vi "Automatic-Approach-Retraction-MCL-2013-04-28-1a-data-storage.vi"() -> ()   [LabVIEW 2012]
uses:
  <vilib>/rvi/eio/common/nirviEmuTemplateMethod_errors.vi
  <vilib>/rvi/Emulation/niFpgaSctlEmulationGetInTimedLoop.vi
  <vilib>/rvi/Emulation/niFpgaSctlEmulationGlobalWrite.vi
  <vilib>/rvi/interface/RandomDataEmulation/nirviRandomDataFPGAFIFO.vi
  <vilib>/rvi/interface/RandomDataEmulation/niFpgaRandomDataHandleErrors.vi
  <vilib>/eio/EIONode/EIONode.xnode
  <vilib>/rvi/Analysis/measure/butterworth/XNode/niFpgaButterworthFilter.xnode
  <vilib>/rvi/DataTransferAndStorage/Container/XNode/niFpgaContainer.xnode
  <vilib>/rvi/interface/RandomDataEmulation/nirviRandomDataFpgaReadWriteTemplate.vi
panel:
  out "Tick Count(Ticks)":u32=3198398528
  in  "Data Acquisition Rate (usec)":u32=500000
  out "Data storage":bool=TRUE
  in  "Safetip Control ON/Off":bool
  out "Start Approach indicator":bool
  in  "safetip time wait":u32 caption="Count(uSec)"
  in  "Safetip retraction":u16
  out "safetip minimum indicator":bool
  out "Data counter":u16
  out "Counter Output":i16
  in  "Initial Position":i16
  in  "phase 1 control":bool
  in  "Manual Control":bool
  in  "Zposition MCL fine 2":i16
  in  "MCL counter 2":u16
  out "Curve indicator":u16
  in  "Number of curves":u16
  out "TF Freq shift":i16
  out "USBS Amplitude":i16
  in  "Timeout FIFO":i32=-1
  in  "Safetip Minimum":i16
  out "Phase 2":bool
  in  "Parameter":i16
  out "Phase 1":bool
  in  "Start Approach":bool
  out "MCL counter in range?":bool
  in  "Wait-tip-before-new-approach (usec)":u32
  in  "Fast Retraction After Cycle":i32
  in  "Wait-tip-before-approach":u32
  in  "Fast Retraction before approach":i32
  in  "Offset for Fast Approach":i16
  in  "Fast Approach (usec)":u32
  out "USBS Phase Signal":i16
  in  "Minimum for Approach Value":i16
  out "digital steps per region":u16
  in  "MCL Divisions":u16
  in  "MCL counter":u16
  in  "Fine Retraction (usec)":u32
  in  "TF at infinity":i16
  out "TF Phase Signal":i16(graph)
  out "Control Signal":i16
  out "MCL Sensor":i16
  in  "Fine Approach (usec)":u32
  in  "Setpoint Fine":i16
  out "Zposition MCL fine":i16
  in  "Initial Height (Fine)":i16=9113
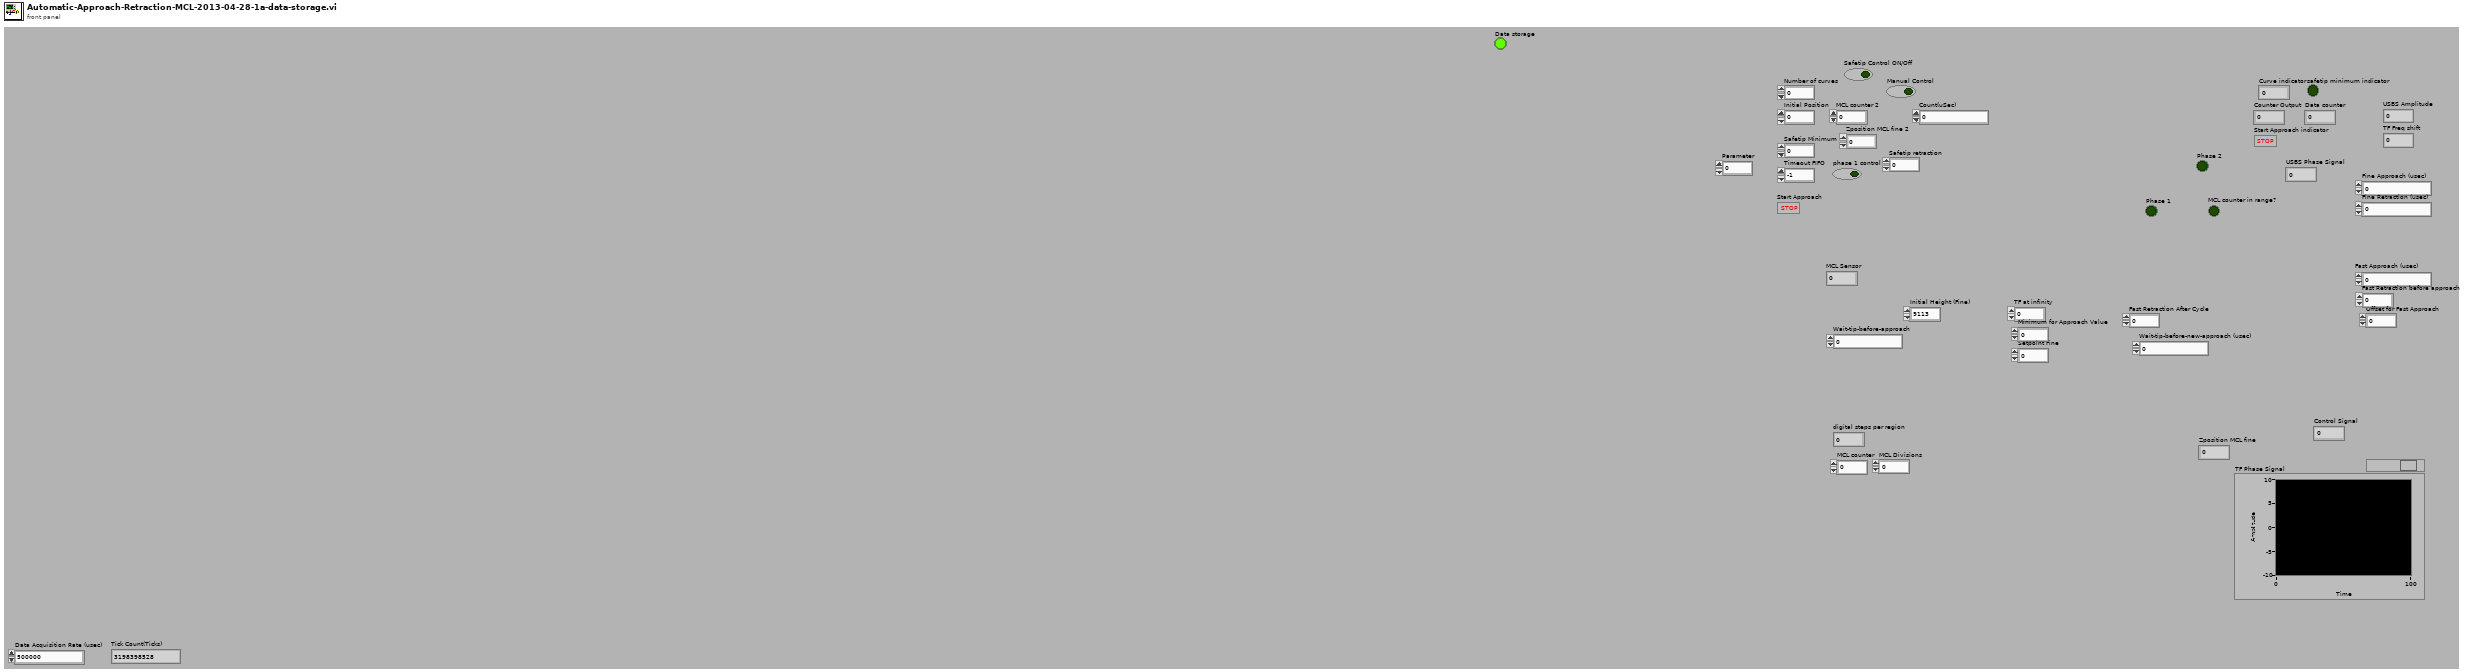
[diagram p1: front panel]
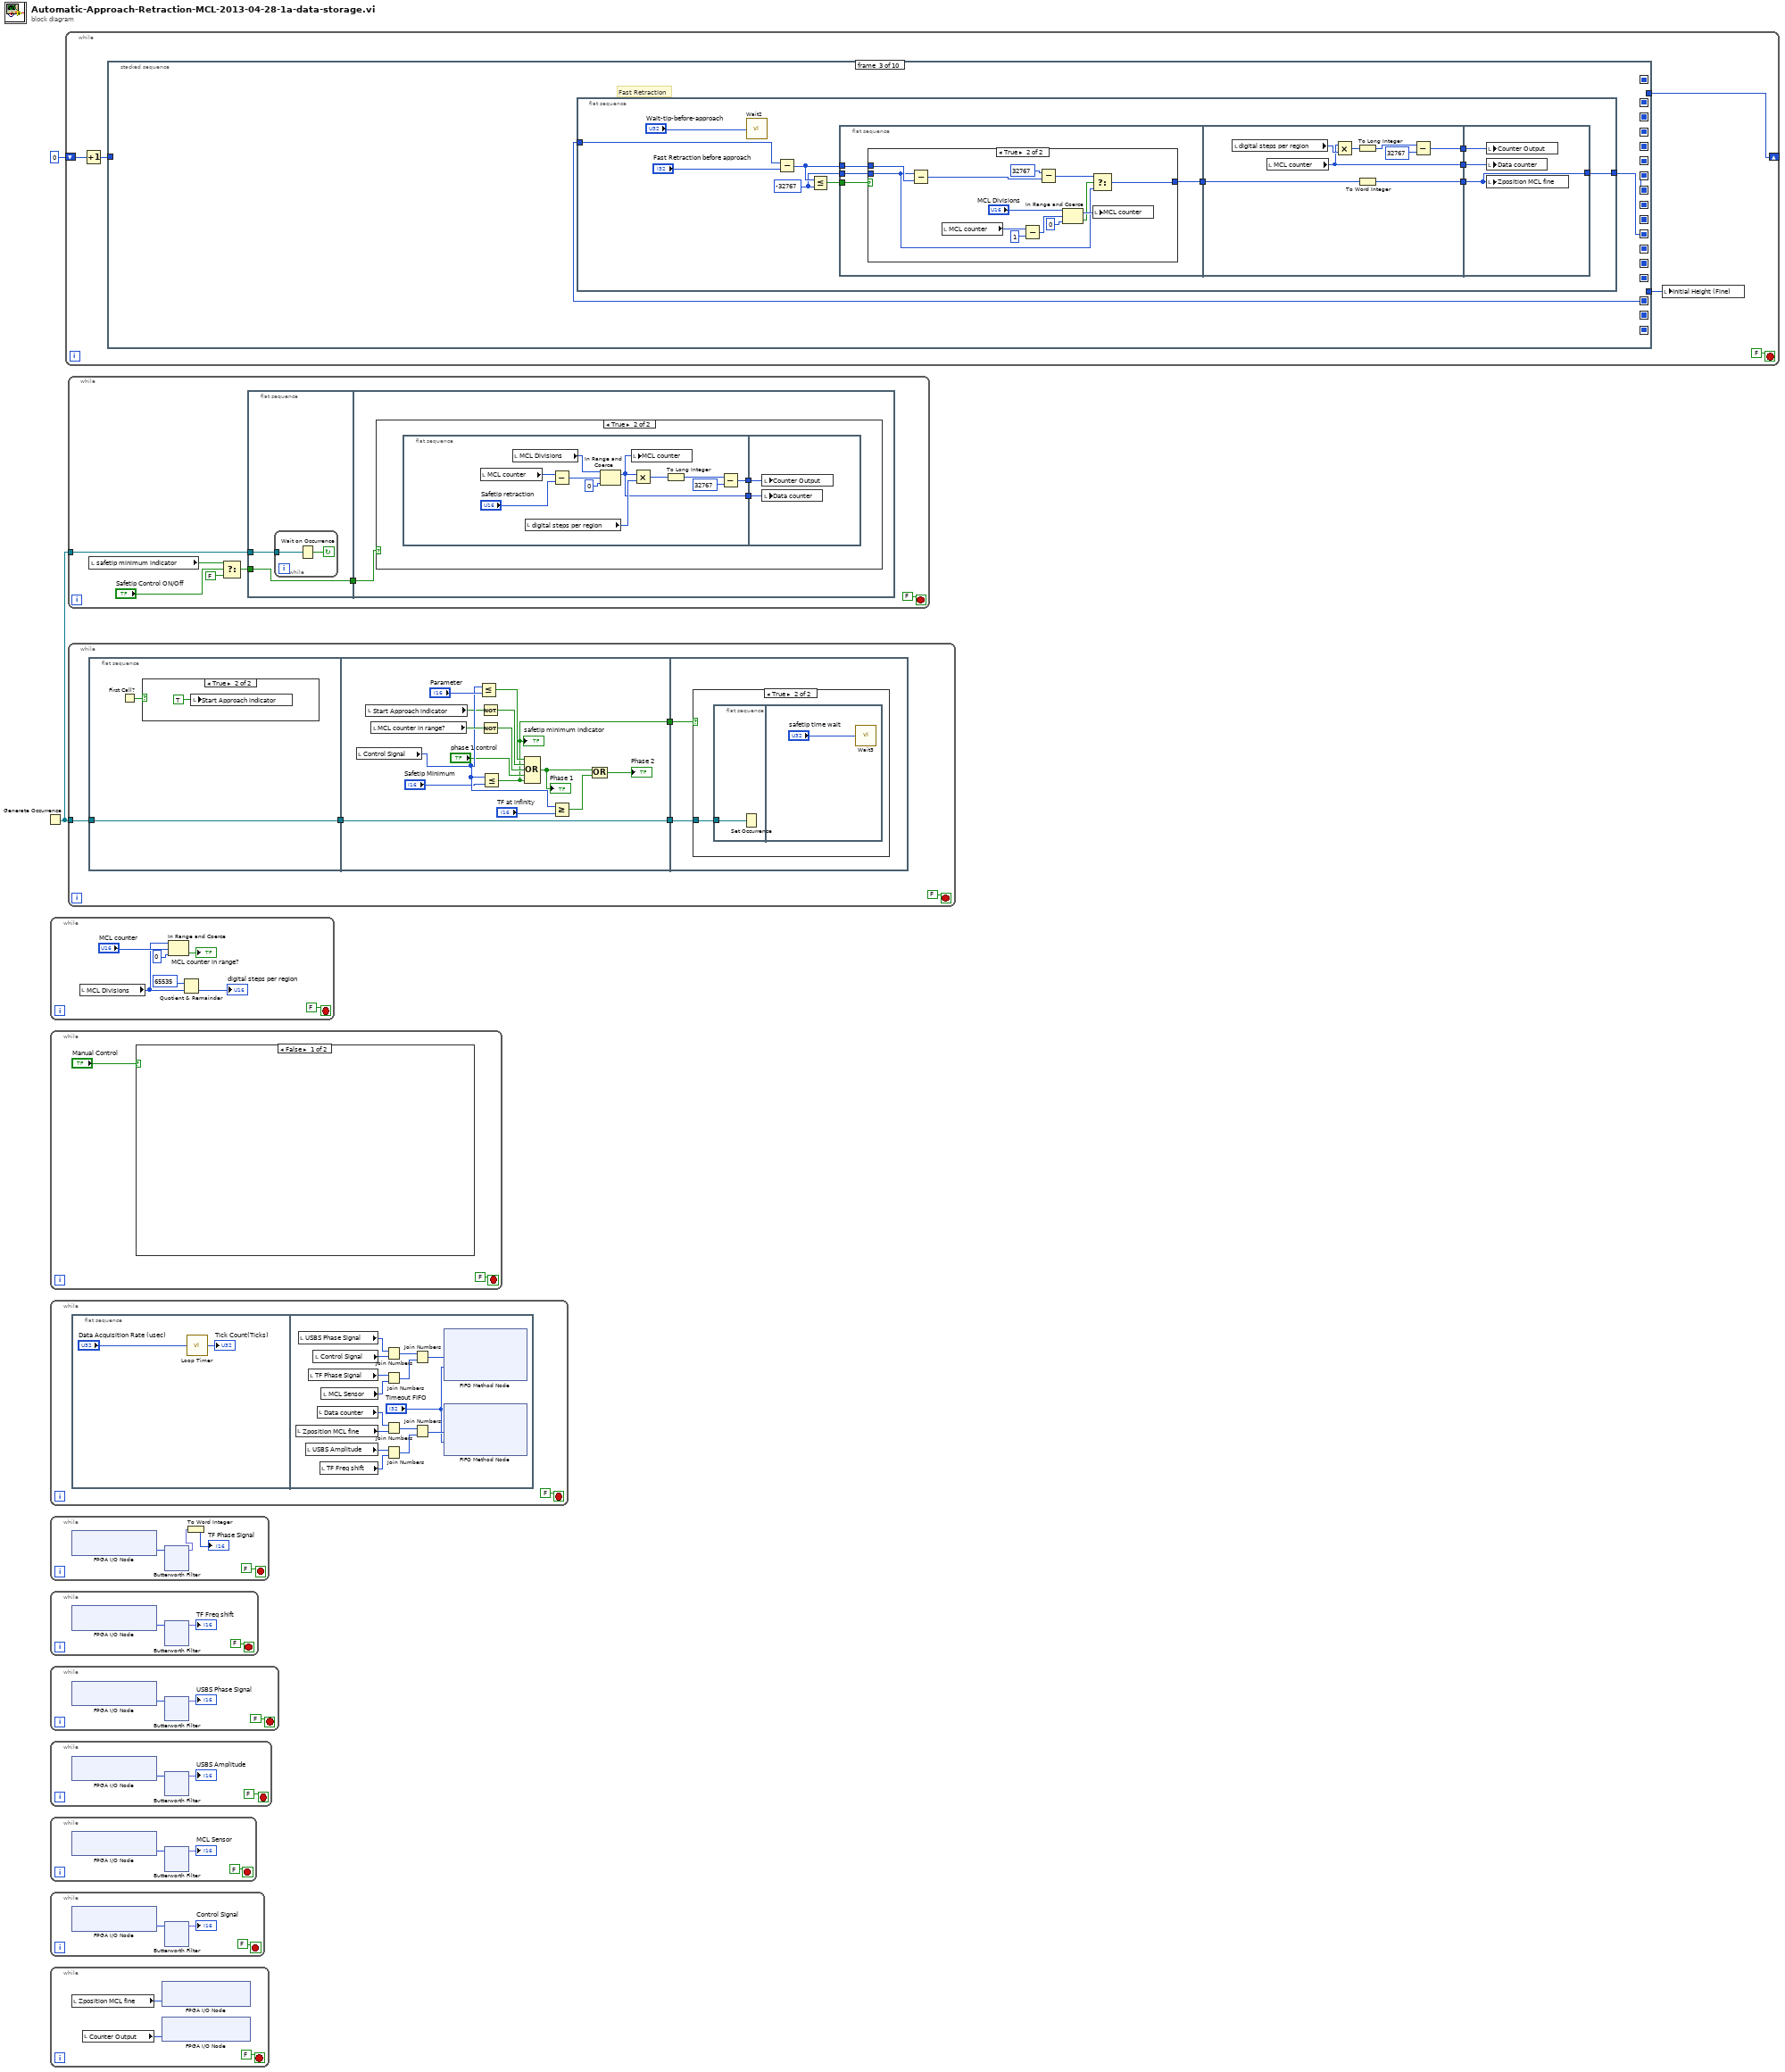
[diagram p0: block diagram]
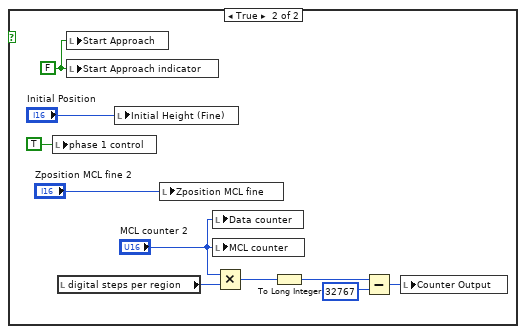
[diagram p3: hidden frame]
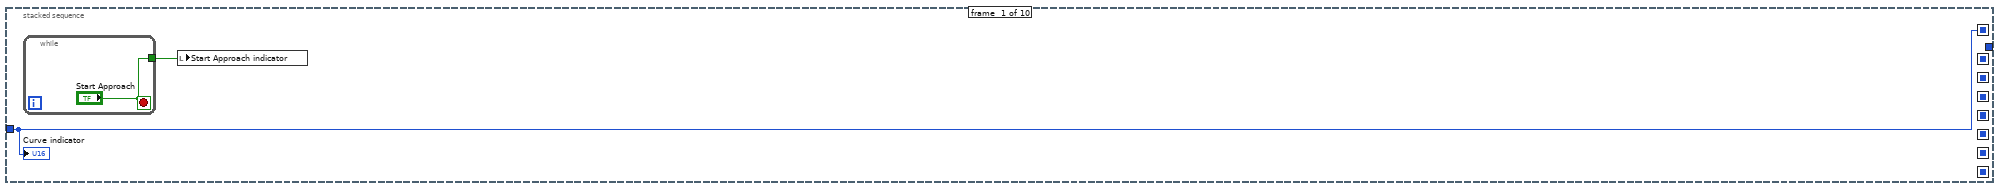
[diagram p6: hidden frame]
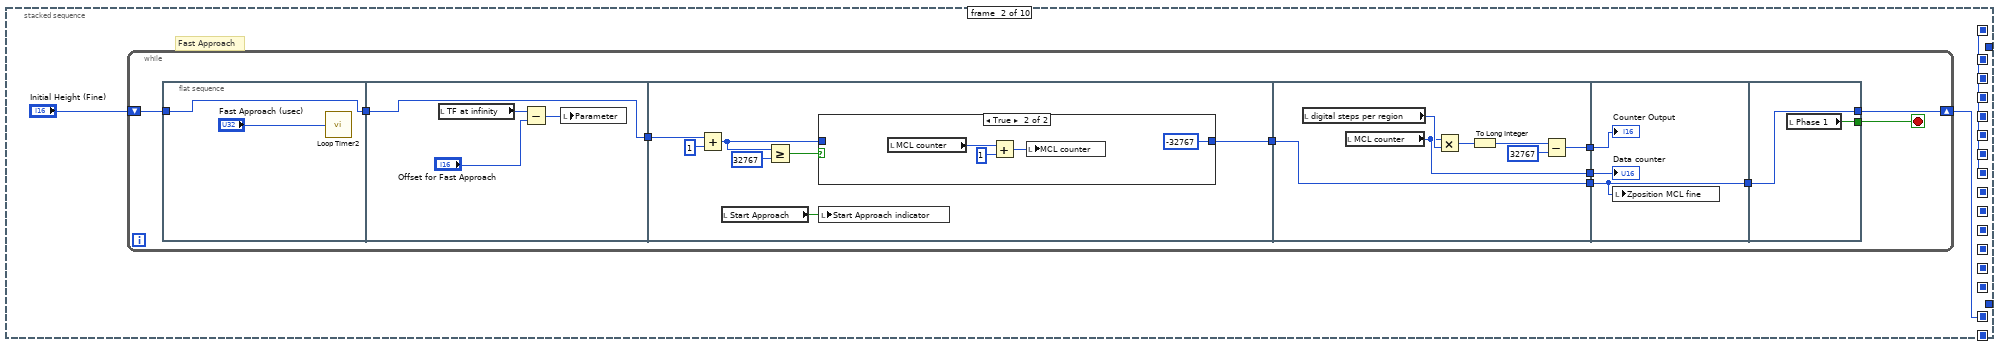
[diagram p7: hidden frame]
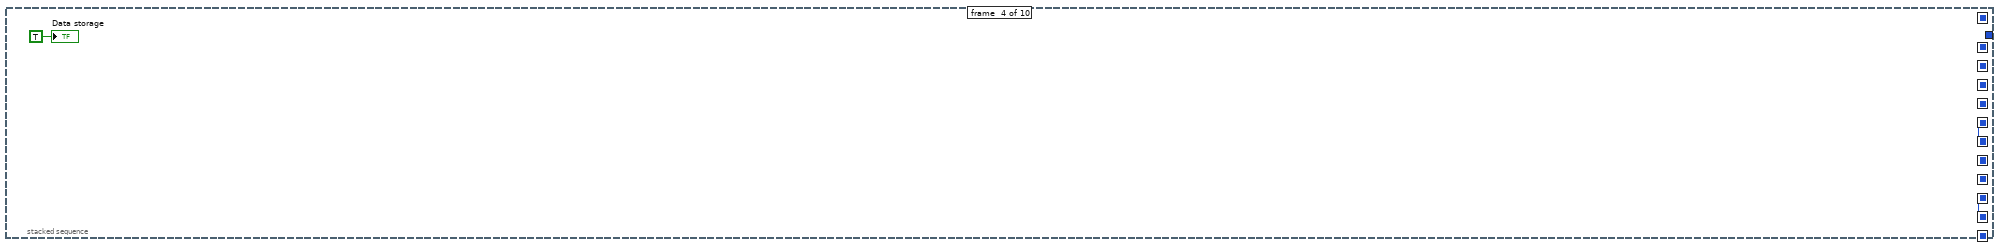
[diagram p10: hidden frame]
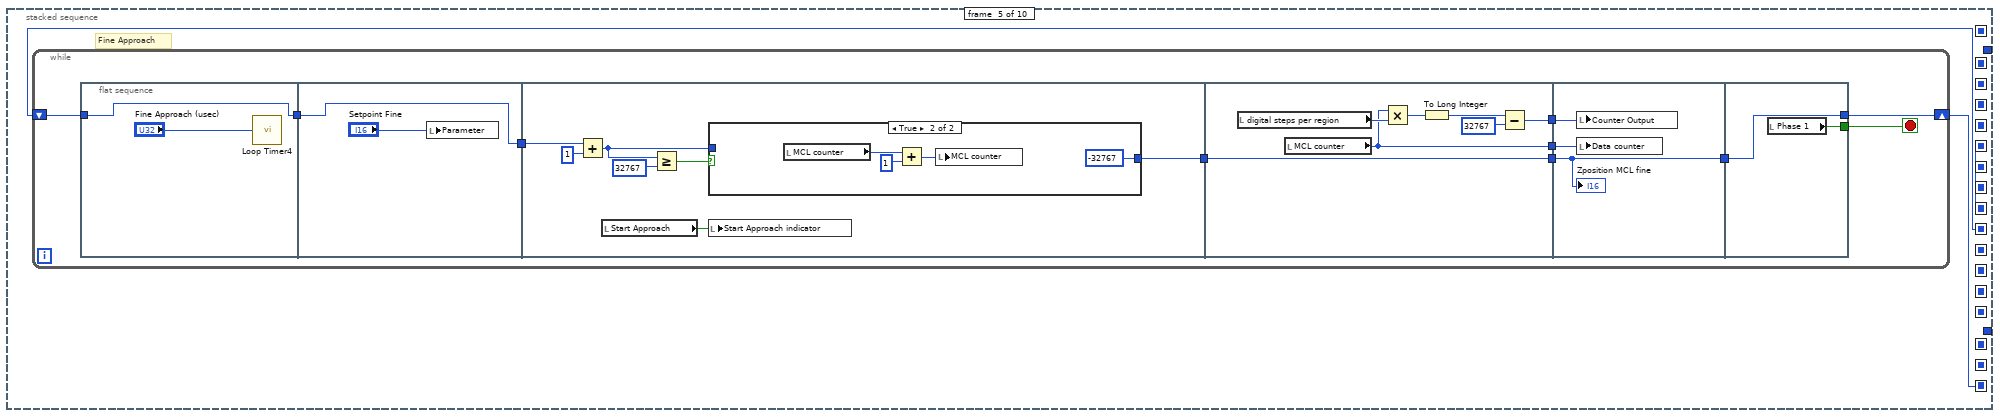
[diagram p11: hidden frame]
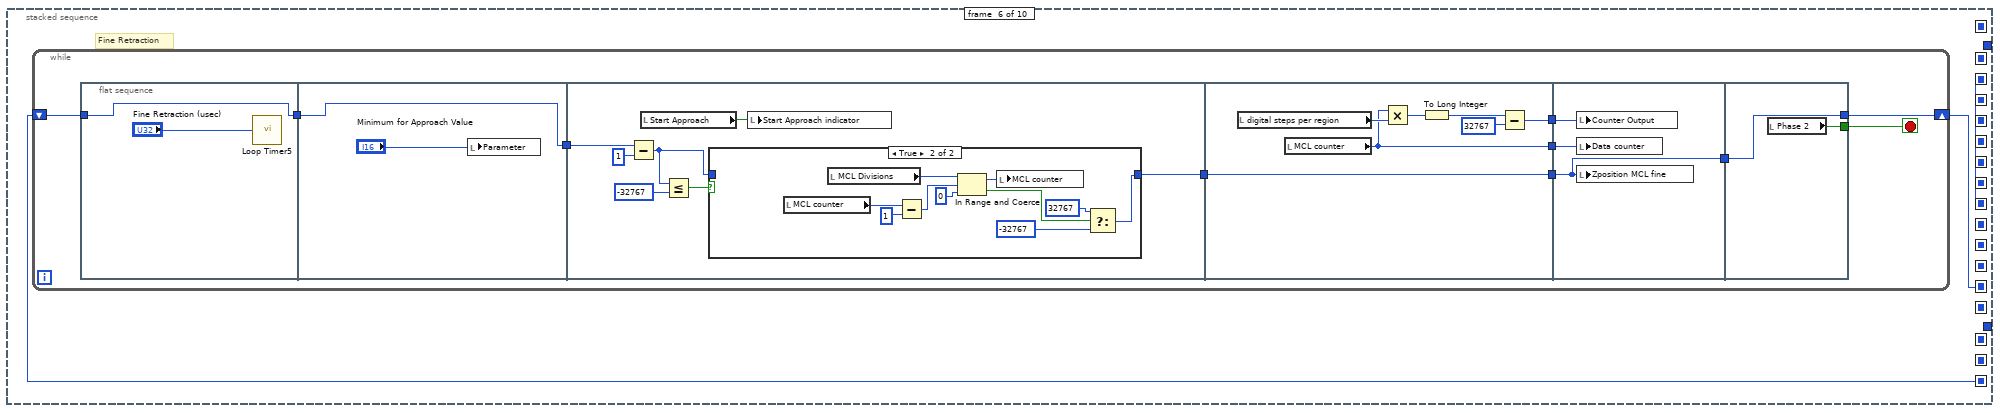
[diagram p13: hidden frame]
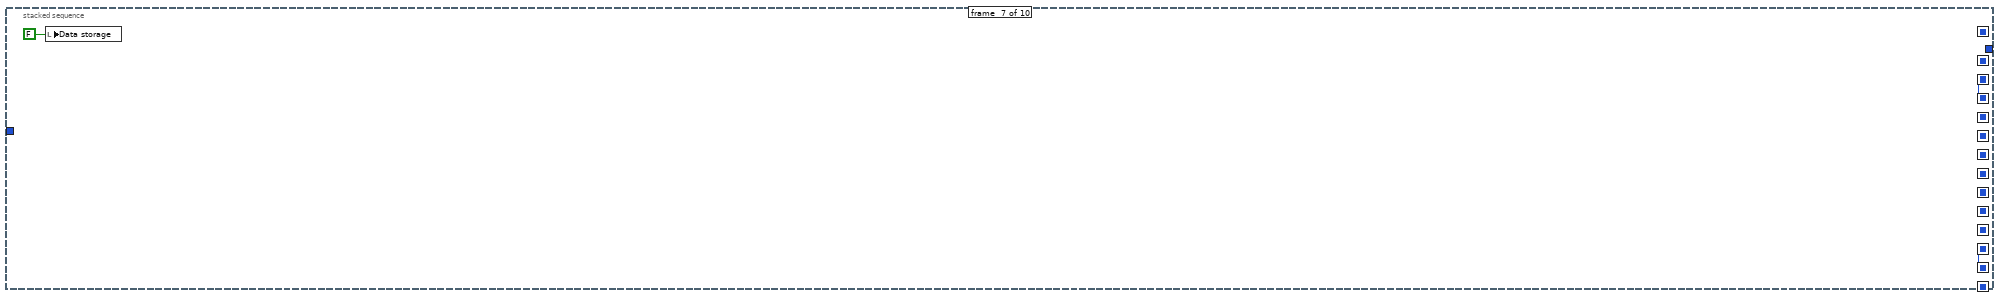
[diagram p15: hidden frame]
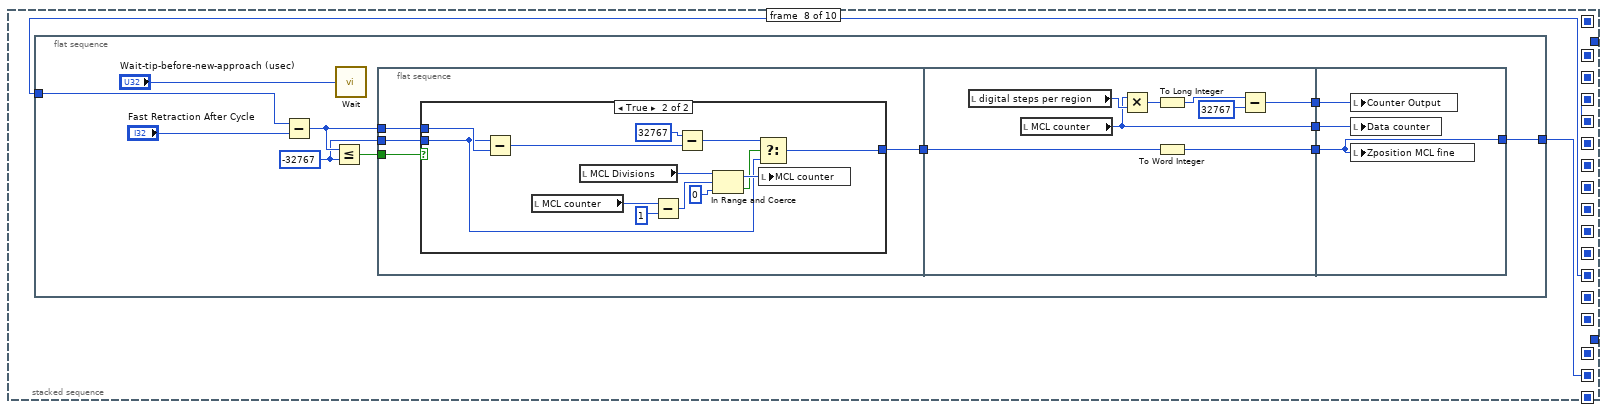
[diagram p16: hidden frame]
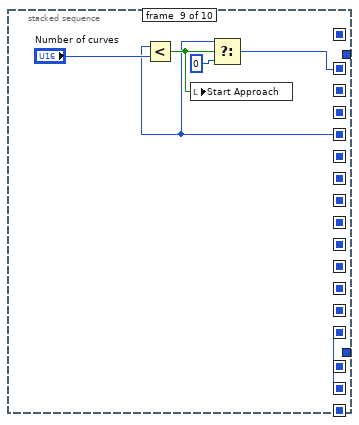
[diagram p18: hidden frame]
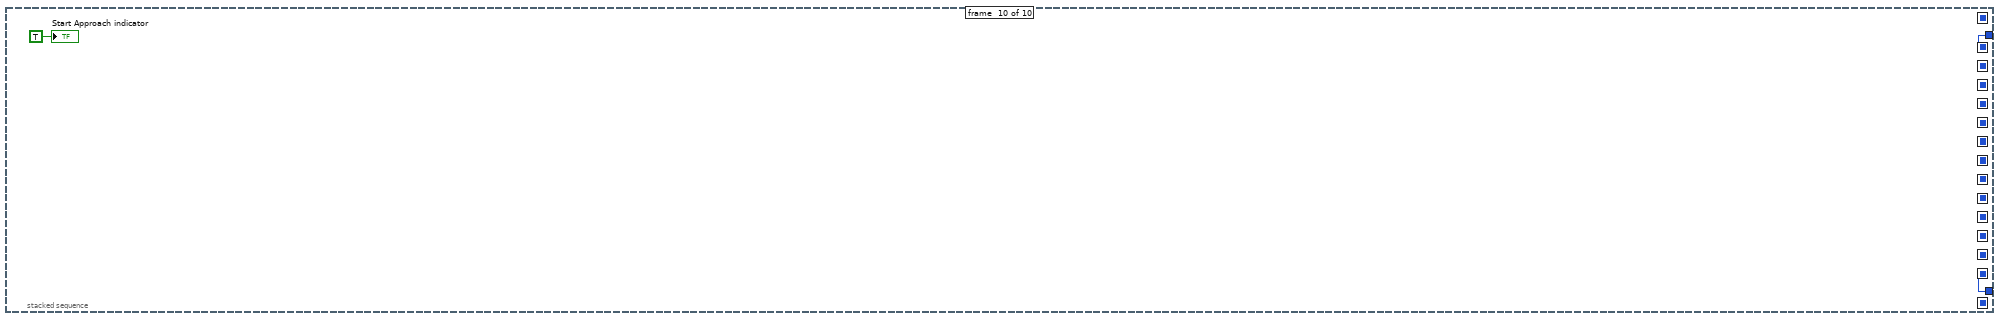
[diagram p19: hidden frame]
diagram:
  n1 = Generate Occurrence() -> (w1:refnum<k4>)
  n2 = while {
    stop <- FALSE stop-if-true
    n3 = local read "MCL Divisions"() -> (w3:u16)
    n4 = In Range and Coerce(upper limit=w3, x="MCL counter", lower limit=u16 0) -> (In Range?=→"MCL counter in range?":bool)  [unwired: 1 out]
    n5 = Quotient & Remainder(x=65535, y=w3) -> (floor(x/y)=→"digital steps per region":i32)  [unwired: 1 out]
  }
  n6 = while {
    stop <- FALSE stop-if-true
    n7 = case shown="False" "Manual Control" {
      frame False {
      }
      frame True {
        w12 = FALSE ("Start Approach")
        n8 = local write "phase 1 control"(TRUE ("phase 1 control")) -> ()
        n9 = local read "digital steps per region"() -> (w18:u16)
        n10 = local write "Start Approach"(w12) -> ()
        n11 = local write "Start Approach indicator"(w12) -> ()
        n12 = local write "Initial Height (Fine)"("Initial Position") -> ()
        n13 = local write "Zposition MCL fine"("Zposition MCL fine 2") -> ()
        n14 = local write "Data counter"("MCL counter 2") -> ()
        n15 = local write "MCL counter"("MCL counter 2") -> ()
        n16 = Multiply(x="MCL counter 2", y=w18) -> (x*y=w14:u16)
        n17 = To Long Integer(number=w14) -> (32bit integer=w13:i32)
        n18 = Subtract(x=w13, y=32767) -> (x-y=w16:i32)
        n19 = local write "Counter Output"(w16) -> ()
      }
    }
  }
  n20 = while {
    stop <- FALSE stop-if-true
    n21 = flat-sequence {
      frame #0 {
        n22 = call "Loop Timer"("Count(Ticks)"="Data Acquisition Rate (usec)") -> ("Tick Count(Ticks)"=→"Tick Count(Ticks)":u32)
      }
      frame #1 {
        n23 = local read "Zposition MCL fine"() -> (w35:i16)
        n24 = local read "USBS Phase Signal"() -> (w30:i16)
        n25 = local read "USBS Amplitude"() -> (w26:i16)
        n26 = local read "TF Phase Signal"() -> (w28:i16)
        n27 = local read "Control Signal"() -> (w29:i16)
        n28 = local read "Data counter"() -> (w36:u16)
        n29 = local read "TF Freq shift"() -> (w25:i16)
        n30 = local read "MCL Sensor"() -> (w27:i16)
        n31 = Join Numbers(hi=w30, lo=w29) -> ((hi.lo)=w38:u32)
        n32 = Join Numbers(hi=w28, lo=w27) -> ((hi.lo)=w39:u32)
        n33 = Join Numbers(hi=w36, lo=w35) -> ((hi.lo)=w33:u32)
        n34 = Join Numbers(hi=w26, lo=w25) -> ((hi.lo)=w34:u32)
        n35 = Join Numbers(hi=w38, lo=w39) -> ((hi.lo)=w37:u64)
        n36 = Join Numbers(hi=w33, lo=w34) -> ((hi.lo)=w32:u64)
        n37 = xnode ("FIFO Method Node")("Element"=w37, "Timeout"="Timeout FIFO") -> ()  [unwired: 1 in, 2 out]
        n38 = xnode ("FIFO Method Node")("Element"=w32, "Timeout"="Timeout FIFO") -> ()  [unwired: 1 in, 2 out]
      }
    }
  }
  n39 = while {
    stop <- FALSE stop-if-true
    n40 = xnode "FPGA I/O Node"() -> ("Connector0/AI1"=w43:i16)  [unwired: 1 in, 1 out]
    n41 = xnode "Butterworth Filter"("input data"=w43) -> ("output data"=w41:fxp<+/-,20,20>)  [unwired: 2 in]
    n42 = To Word Integer(number=w41) -> (16bit integer=→"TF Phase Signal":i16)
  }
  n43 = while {
    stop <- FALSE stop-if-true
    n44 = xnode "FPGA I/O Node"() -> ("Connector0/AI2"=w53:i16)  [unwired: 1 in, 1 out]
    n45 = xnode "Butterworth Filter"("input data"=w53) -> ("output data"=→"TF Freq shift":fxp<+/-,20,20>)  [unwired: 2 in]
  }
  n46 = while {
    stop <- FALSE stop-if-true
    n47 = xnode "FPGA I/O Node"() -> ("Connector0/AI4"=w63:i16)  [unwired: 1 in, 1 out]
    n48 = xnode "Butterworth Filter"("input data"=w63) -> ("output data"=→"USBS Phase Signal":fxp<+/-,20,20>)  [unwired: 2 in]
  }
  n49 = while {
    stop <- FALSE stop-if-true
    n50 = xnode "FPGA I/O Node"() -> ("Connector0/AI5"=w73:i16)  [unwired: 1 in, 1 out]
    n51 = xnode "Butterworth Filter"("input data"=w73) -> ("output data"=→"USBS Amplitude":fxp<+/-,20,20>)  [unwired: 2 in]
  }
  n52 = while {
    stop <- FALSE stop-if-true
    n53 = xnode "FPGA I/O Node"() -> ("Connector0/AI6"=w83:i16)  [unwired: 1 in, 1 out]
    n54 = xnode "Butterworth Filter"("input data"=w83) -> ("output data"=→"MCL Sensor":fxp<+/-,20,20>)  [unwired: 2 in]
  }
  n55 = while {
    stop <- FALSE stop-if-true
    n56 = xnode "FPGA I/O Node"() -> ("Connector0/AI7"=w93:i16)  [unwired: 1 in, 1 out]
    n57 = xnode "Butterworth Filter"("input data"=w93) -> ("output data"=→"Control Signal":fxp<+/-,20,20>)  [unwired: 2 in]
  }
  n58 = while {
    stop <- FALSE stop-if-true
    n59 = local read "Zposition MCL fine"() -> (w102:i16)
    n60 = local read "Counter Output"() -> (w101:i16)
    n61 = xnode "FPGA I/O Node"("Connector0/AO7"=w102) -> ()  [unwired: 1 in, 1 out]
    n62 = xnode "FPGA I/O Node"("Connector0/AO2"=w101) -> ()  [unwired: 1 in, 1 out]
  }
  n63 = while {
    shift-right: [w105] -> _
    shift-left: u16 0 ("t") -> [w104]
    stop <- FALSE stop-if-true
    n64 = Increment(x=w104) -> (x+1=w106:u16)
    n65 = stacked-sequence {
      seq-local: [w110 _ _ _ _ _ _ _ _ _] -> [_ w113 _ _ _ _ _ _ _ _]
      seq-local: [_ w114 _ _ _ _ _ _ _ _] -> [_ _ w157 _ _ _ _ _ _ _]
      seq-local: [_ w113 _ _ _ _ _ _ _ _] -> [_ _ w155 _ _ _ _ _ _ _]
      seq-local: [_ _ w156 _ _ _ _ _ _ _] -> [_ _ _ w200 _ _ _ _ _ _]
      seq-local: [_ _ w155 _ _ _ _ _ _ _] -> [_ _ _ w199 _ _ _ _ _ _]
      seq-local: [_ _ _ w200 _ _ _ _ _ _] -> [_ _ _ _ w203 _ _ _ _ _]
      seq-local: [_ _ _ w199 _ _ _ _ _ _] -> [_ _ _ _ w201 _ _ _ _ _]
      seq-local: [_ _ _ _ w202 _ _ _ _ _] -> [_ _ _ _ _ w244 _ _ _ _]
      seq-local: [_ _ _ _ w201 _ _ _ _ _] -> [_ _ _ _ _ w242 _ _ _ _]
      seq-local: [_ _ _ _ _ w243 _ _ _ _] -> [_ _ _ _ _ _ w291 _ _ _]
      seq-local: [_ _ _ _ _ w242 _ _ _ _] -> [_ _ _ _ _ _ w290 _ _ _]
      seq-local: [_ _ _ _ _ _ w291 _ _ _] -> [_ _ _ _ _ _ _ w294 _ _]
      seq-local: [_ _ _ _ _ _ w290 _ _ _] -> [_ _ _ _ _ _ _ w292 _ _]
      seq-local: [_ _ _ _ _ _ _ w293 _ _] -> [_ _ _ _ _ _ _ _ w340 _]
      seq-local: [_ _ _ _ _ _ _ w292 _ _] -> [_ _ _ _ _ _ _ _ w335 _]
      seq-local: [_ _ _ _ _ _ _ _ w340 _] -> [_ _ _ _ _ _ _ _ _ w343]
      seq-local: [_ _ _ _ _ _ _ _ w336 _] -> [_ _ _ _ _ _ _ _ _ w342]
      tunnel: w106 -> [w110 _ _ _ _ _ _ _ _ _]
      tunnel: [_ _ _ _ _ _ _ _ _ w343] -> w108
      tunnel: [_ _ _ _ _ _ _ _ _ w342] -> w105
      frame #0 {
        n66 = while {
          tunnel: ["Start Approach"] -> w109
          stop <- "Start Approach" stop-if-true
        }
        n67 = local write "Start Approach indicator"(w109) -> ()
        "Curve indicator" <- w110
      }
      frame #1 {
        # "Fast Approach"
        n68 = while {
          shift-right: [w123] -> w114
          shift-left: "Initial Height (Fine)" -> [w124]
          stop <- w119 stop-if-true
          n69 = flat-sequence {
            tunnel: w124 -> [w126]
            tunnel: [w126] -> w121
            tunnel: [w130] -> w122
            tunnel: w121 -> [w130]
            tunnel: [w136] -> w118
            tunnel: w122 -> [w137]
            tunnel: w118 -> [w149]
            tunnel: [w149] -> w117
            tunnel: [w146] -> w116
            tunnel: [w145] -> w115
            tunnel: w117 -> [w152]
            tunnel: [w152] -> w120
            tunnel: w116 -> [w151]
            tunnel: w115 -> [w150]
            tunnel: [w154] -> w123
            tunnel: w120 -> [w154]
            tunnel: [w153] -> w119
            frame #0 {
              n70 = call "Loop Timer2"("Count(uSec)"="Fast Approach (usec)") -> ()  [unwired: 1 out]
            }
            frame #1 {
              n71 = local read "TF at infinity"() -> (w127:i16)
              n72 = Subtract(x=w127, y="Offset for Fast Approach") -> (x-y=w129:i16)
              n73 = local write "Parameter"(w129) -> ()
            }
            frame #2 {
              n74 = Add(x=w137, y=i16 1) -> (x+y=w132:i16)
              n75 = local read "Start Approach"() -> (w131:bool)
              n76 = Greater Or Equal?(x=w132, y=i16 32767) -> (x >= y?=w133:bool)
              n77 = case shown="True" w133 {
                tunnel: [w138 i16 -32767] -> w136
                tunnel: w132 -> [w138 _]
                frame False {
                }
                frame True {
                  n78 = local read "MCL counter"() -> (w140:u16)
                  n79 = Add(x=w140, y=u16 1) -> (x+y=w139:u16)
                  n80 = local write "MCL counter"(w139) -> ()
                }
              }
              n81 = local write "Start Approach indicator"(w131) -> ()
            }
            frame #3 {
              n82 = local read "digital steps per region"() -> (w148:u16)
              n83 = local read "MCL counter"() -> (w145:u16)
              n84 = Multiply(x=w145, y=w148) -> (x*y=w144:u16)
              n85 = To Long Integer(number=w144) -> (32bit integer=w143:i32)
              n86 = Subtract(x=w143, y=32767) -> (x-y=w146:i32)
            }
            frame #4 {
              n87 = local write "Zposition MCL fine"(w152) -> ()
              "Counter Output" <- w151
              "Data counter" <- w150
            }
            frame #5 {
              n88 = local read "Phase 1"() -> (w153:bool)
            }
          }
        }
      }
      frame #2 {
        # "Fast Retraction"
        n89 = flat-sequence {
          tunnel: [w164] -> w156
          tunnel: w157 -> [w165]
          frame #0 {
            w162 = -32767 ("y")
            n90 = call "Wait2"("Count(uSec)"="Wait-tip-before-approach") -> ()  [unwired: 1 out]
            n91 = Subtract(x=w165, y="Fast Retraction before approach") -> (x-y=w167:i32)
            n92 = Less Or Equal?(x=w167, y=w162) -> (x <= y?=w168:bool)
            n93 = flat-sequence {
              tunnel: w168 -> [w172]
              tunnel: w167 -> [w171]
              tunnel: w162 -> [w169]
              tunnel: [w170] -> w161
              tunnel: w161 -> [w190]
              tunnel: [w189] -> w160
              tunnel: [w191] -> w159
              tunnel: [w192] -> w158
              tunnel: [w197] -> w164
              tunnel: w160 -> [w197]
              tunnel: w159 -> [w196]
              tunnel: w158 -> [w195]
              frame #0 {
                n94 = case shown="True" w172 {
                  tunnel: w171 -> [w173 w183]
                  tunnel: [w173 w175] -> w170
                  tunnel: w169 -> [_ w174]
                  frame False {
                  }
                  frame True {
                    n95 = Subtract(x=w174, y=w183) -> (x-y=w182:i32)
                    n96 = local read "MCL counter"() -> (w186:u16)
                    n97 = Subtract(x=w186, y=u16 1) -> (x-y=w179:u16)
                    n98 = Subtract(x=32767, y=w182) -> (x-y=w176:i32)
                    n99 = In Range and Coerce(upper limit="MCL Divisions", x=w179, lower limit=u16 0 ("upper limit")) -> (coerced(x)=w178:u16, In Range?=w177:bool)
                    n100 = Select(t=w176, s=w177, f=w174) -> (s? t:f=w175:i32)
                    n101 = local write "MCL counter"(w178) -> ()
                  }
                }
              }
              frame #1 {
                n102 = local read "digital steps per region"() -> (w194:u16)
                n103 = local read "MCL counter"() -> (w191:u16)
                n104 = Multiply(x=w191, y=w194) -> (x*y=w188:u16)
                n105 = To Long Integer(number=w188) -> (32bit integer=w187:i32)
                n106 = To Word Integer(number=w190) -> (16bit integer=w189:i16)
                n107 = Subtract(x=w187, y=32767) -> (x-y=w192:i32)
              }
              frame #2 {
                n108 = local write "Counter Output"(w195) -> ()
                n109 = local write "Data counter"(w196) -> ()
                n110 = local write "Zposition MCL fine"(w197) -> ()
              }
            }
          }
        }
      }
      frame #3 {
        "Data storage" <- TRUE
      }
      frame #4 {
        # "Fine Approach"
        n111 = while {
          shift-right: [w212] -> w202
          shift-left: w203 -> [w213]
          stop <- w204 stop-if-true
          n112 = flat-sequence {
            tunnel: w213 -> [w215]
            tunnel: [w215] -> w210
            tunnel: [w217] -> w211
            tunnel: w210 -> [w217]
            tunnel: [w223] -> w209
            tunnel: w211 -> [w224]
            tunnel: w209 -> [w236]
            tunnel: [w236] -> w208
            tunnel: [w233] -> w207
            tunnel: [w232] -> w206
            tunnel: w208 -> [w237]
            tunnel: w207 -> [w239]
            tunnel: w206 -> [w238]
            tunnel: [w237] -> w205
            tunnel: [w241] -> w212
            tunnel: w205 -> [w241]
            tunnel: [w240] -> w204
            frame #0 {
              n113 = call "Loop Timer4"("Count(uSec)"="Fine Approach (usec)") -> ()  [unwired: 1 out]
            }
            frame #1 {
              n114 = local write "Parameter"("Setpoint Fine") -> ()
            }
            frame #2 {
              n115 = Add(x=w224, y=i16 1) -> (x+y=w219:i16)
              n116 = local read "Start Approach"() -> (w218:bool)
              n117 = Greater Or Equal?(x=w219, y=i16 32767) -> (x >= y?=w220:bool)
              n118 = case shown="True" w220 {
                tunnel: [w225 i16 -32767] -> w223
                tunnel: w219 -> [w225 _]
                frame False {
                }
                frame True {
                  n119 = local read "MCL counter"() -> (w226:u16)
                  n120 = Add(x=w226, y=u16 1) -> (x+y=w228:u16)
                  n121 = local write "MCL counter"(w228) -> ()
                }
              }
              n122 = local write "Start Approach indicator"(w218) -> ()
            }
            frame #3 {
              n123 = local read "digital steps per region"() -> (w235:u16)
              n124 = local read "MCL counter"() -> (w232:u16)
              n125 = Multiply(x=w232, y=w235) -> (x*y=w231:u16)
              n126 = To Long Integer(number=w231) -> (32bit integer=w230:i32)
              n127 = Subtract(x=w230, y=32767) -> (x-y=w233:i32)
            }
            frame #4 {
              n128 = local write "Counter Output"(w239) -> ()
              n129 = local write "Data counter"(w238) -> ()
              "Zposition MCL fine" <- w237
            }
            frame #5 {
              n130 = local read "Phase 1"() -> (w240:bool)
            }
          }
        }
      }
      frame #5 {
        # "Fine Retraction"
        n131 = while {
          shift-right: [w253] -> w243
          shift-left: w244 -> [w254]
          stop <- w247 stop-if-true
          n132 = flat-sequence {
            tunnel: w254 -> [w256]
            tunnel: [w256] -> w250
            tunnel: [w258] -> w251
            tunnel: w250 -> [w258]
            tunnel: [w264] -> w252
            tunnel: w251 -> [w265]
            tunnel: w252 -> [w283]
            tunnel: [w283] -> w249
            tunnel: [w278] -> w246
            tunnel: [w277] -> w245
            tunnel: w249 -> [w284]
            tunnel: [w284] -> w248
            tunnel: w246 -> [w286]
            tunnel: w245 -> [w285]
            tunnel: [w288] -> w253
            tunnel: w248 -> [w288]
            tunnel: [w287] -> w247
            frame #0 {
              n133 = call "Loop Timer5"("Count(uSec)"="Fine Retraction (usec)") -> ()  [unwired: 1 out]
            }
            frame #1 {
              n134 = local write "Parameter"("Minimum for Approach Value") -> ()
            }
            frame #2 {
              n135 = Subtract(x=w265, y=i16 1) -> (x-y=w260:i16)
              n136 = local read "Start Approach"() -> (w259:bool)
              n137 = Less Or Equal?(x=w260, y=i16 -32767) -> (x <= y?=w262:bool)
              n138 = case shown="True" w262 {
                tunnel: w260 -> [w266 _]
                tunnel: [w266 w267] -> w264
                frame False {
                }
                frame True {
                  n139 = local read "MCL counter"() -> (w276:u16)
                  n140 = local read "MCL Divisions"() -> (w274:u16)
                  n141 = Subtract(x=w276, y=u16 1) -> (x-y=w272:u16)
                  n142 = In Range and Coerce(upper limit=w274, x=w272, lower limit=u16 0) -> (coerced(x)=w271:u16, In Range?=w270:bool)
                  n143 = local write "MCL counter"(w271) -> ()
                  n144 = Select(t=i16 32767, s=w270, f=i16 -32767) -> (s? t:f=w267:i16)
                }
              }
              n145 = local write "Start Approach indicator"(w259) -> ()
            }
            frame #3 {
              n146 = local read "digital steps per region"() -> (w282:u16)
              n147 = local read "MCL counter"() -> (w278:u16)
              n148 = Multiply(x=w278, y=w282) -> (x*y=w280:u16)
              n149 = To Long Integer(number=w280) -> (32bit integer=w279:i32)
              n150 = Subtract(x=w279, y=32767) -> (x-y=w277:i32)
            }
            frame #4 {
              n151 = local write "Counter Output"(w285) -> ()
              n152 = local write "Data counter"(w286) -> ()
              n153 = local write "Zposition MCL fine"(w284) -> ()
            }
            frame #5 {
              n154 = local read "Phase 2"() -> (w287:bool)
            }
          }
        }
      }
      frame #6 {
        n155 = local write "Data storage"(FALSE ("Data storage")) -> ()
      }
      frame #7 {
        n156 = flat-sequence {
          tunnel: [w301] -> w293
          tunnel: w294 -> [w302]
          frame #0 {
            w299 = -32767 ("y")
            n157 = Subtract(x=w302, y="Fast Retraction After Cycle") -> (x-y=w305:i32)
            n158 = Less Or Equal?(x=w305, y=w299) -> (x <= y?=w304:bool)
            n159 = call "Wait"("Count(uSec)"="Wait-tip-before-new-approach (usec)") -> ()  [unwired: 1 out]
            n160 = flat-sequence {
              tunnel: w305 -> [w309]
              tunnel: w304 -> [w308]
              tunnel: w299 -> [w306]
              tunnel: [w307] -> w298
              tunnel: w298 -> [w327]
              tunnel: [w326] -> w297
              tunnel: [w329] -> w296
              tunnel: [w328] -> w295
              tunnel: [w333] -> w301
              tunnel: w297 -> [w333]
              tunnel: w296 -> [w334]
              tunnel: w295 -> [w332]
              frame #0 {
                n161 = case shown="True" w308 {
                  tunnel: w309 -> [w310 w321]
                  tunnel: [w310 w311] -> w307
                  tunnel: w306 -> [_ w312]
                  frame False {
                  }
                  frame True {
                    n162 = Subtract(x=w312, y=w321) -> (x-y=w320:i32)
                    n163 = local read "MCL counter"() -> (w323:u16)
                    n164 = local read "MCL Divisions"() -> (w317:u16)
                    n165 = Subtract(x=w323, y=u16 1) -> (x-y=w318:u16)
                    n166 = Subtract(x=32767, y=w320) -> (x-y=w313:i32)
                    n167 = In Range and Coerce(upper limit=w317, x=w318, lower limit=u16 0) -> (coerced(x)=w315:u16, In Range?=w314:bool)
                    n168 = Select(t=w313, s=w314, f=w312) -> (s? t:f=w311:i32)
                    n169 = local write "MCL counter"(w315) -> ()
                  }
                }
              }
              frame #1 {
                n170 = local read "digital steps per region"() -> (w331:u16)
                n171 = local read "MCL counter"() -> (w328:u16)
                n172 = Multiply(x=w328, y=w331) -> (x*y=w325:u16)
                n173 = To Long Integer(number=w325) -> (32bit integer=w324:i32)
                n174 = To Word Integer(number=w327) -> (16bit integer=w326:i16)
                n175 = Subtract(x=w324, y=32767) -> (x-y=w329:i32)
              }
              frame #2 {
                n176 = local write "Counter Output"(w334) -> ()
                n177 = local write "Data counter"(w332) -> ()
                n178 = local write "Zposition MCL fine"(w333) -> ()
              }
            }
          }
        }
      }
      frame #8 {
        n179 = Less?(x=w335, y="Number of curves") -> (x < y?=w338:bool)
        n180 = local write "Start Approach"(w338) -> ()
        n181 = Select(t=w335, s=w338, f=u16 0 ("t")) -> (s? t:f=w336:u16)
      }
      frame #9 {
        "Start Approach indicator" <- TRUE ("Start Approach indicator")
      }
    }
    n182 = local write "Initial Height (Fine)"(w108) -> ()
  }
  n183 = while {
    tunnel: w1 -> [w346]
    stop <- FALSE stop-if-true
    n184 = local read "safetip minimum indicator"() -> (w349:bool)
    n185 = Select(t=w349, s="Safetip Control ON/Off", f=FALSE) -> (s? t:f=w344:bool)
    n186 = flat-sequence {
      tunnel: w346 -> [w352]
      tunnel: [w351] -> w345
      tunnel: w344 -> [w351]
      tunnel: w345 -> [w355]
      frame #0 {
        n187 = while {
          tunnel: w352 -> [w353]
          stop <- w354 continue-if-true
          n188 = Wait on Occurrence(2:w353) -> (0:w354:bool)  [unwired: 2 in]
        }
      }
      frame #1 {
        n189 = case shown="True" w355 {
          frame False {
          }
          frame True {
            n190 = flat-sequence {
              tunnel: [w362] -> w357
              tunnel: [w358] -> w356
              tunnel: w357 -> [w370]
              tunnel: w356 -> [w369]
              frame #0 {
                n191 = local read "MCL counter"() -> (w366:u16)
                n192 = local read "MCL Divisions"() -> (w365:u16)
                n193 = local read "digital steps per region"() -> (w368:u16)
                n194 = Subtract(x=w366, y="Safetip retraction") -> (x-y=w363:u16)
                n195 = In Range and Coerce(upper limit=w365, x=w363, lower limit=u16 0) -> (coerced(x)=w362:u16)  [unwired: 1 out]
                n196 = local write "MCL counter"(w362) -> ()
                n197 = Multiply(x=w362, y=w368) -> (x*y=w361:u16)
                n198 = To Long Integer(number=w361) -> (32bit integer=w360:i32)
                n199 = Subtract(x=w360, y=32767) -> (x-y=w358:i32)
              }
              frame #1 {
                n200 = local write "Counter Output"(w369) -> ()
                n201 = local write "Data counter"(w370) -> ()
              }
            }
          }
        }
      }
    }
  }
  n202 = while {
    tunnel: w1 -> [w373]
    stop <- FALSE stop-if-true
    n203 = flat-sequence {
      tunnel: [w376] -> w374
      tunnel: w373 -> [w376]
      tunnel: [w381] -> w372
      tunnel: w374 -> [w379]
      tunnel: [w379] -> w371
      tunnel: w372 -> [w395]
      tunnel: w371 -> [w394]
      frame #0 {
        n204 = First Call?() -> (First Call?: T/F=w377:bool)
        n205 = case shown="True" w377 {
          frame False {
          }
          frame True {
            n206 = local write "Start Approach indicator"(TRUE ("Start Approach indicator")) -> ()
          }
        }
      }
      frame #1 {
        n207 = local read "Control Signal"() -> (w385:i16)
        n208 = local read "Start Approach indicator"() -> (w380:bool)
        n209 = local read "MCL counter in range?"() -> (w392:bool)
        n210 = Less Or Equal?(x=w385, y="Parameter") -> (x <= y?=w390:bool)
        n211 = Not(x=w380) -> (.not. x?=w391:bool)
        n212 = Not(x=w392) -> (.not. x?=w393:bool)
        n213 = Less Or Equal?(x=w385, y="Safetip Minimum") -> (x <= y?=w381:bool)
        "safetip minimum indicator" <- w381
        n214 = Compound Arithmetic op=OR(w390, w391, w393, "phase 1 control", w381) -> (w382:bool)
        "Phase 1" <- w382
        n215 = Greater Or Equal?(x=w385, y="TF at infinity") -> (x >= y?=w387:bool)
        n216 = Compound Arithmetic op=OR(w382, w387) -> (→"Phase 2":bool)
      }
      frame #2 {
        n217 = case shown="True" w395 {
          tunnel: w394 -> [_ w396]
          frame False {
          }
          frame True {
            n218 = flat-sequence {
              tunnel: w396 -> [w397]
              frame #0 {
                n219 = Set Occurrence(w397) -> ()
              }
              frame #1 {
                n220 = call "Wait3"("Count(uSec)"="safetip time wait") -> ()  [unwired: 1 out]
              }
            }
          }
        }
      }
    }
  }
